vi "RSZVB Start Calibration.vi"(6 "Port 1 (1)":i32=1, 7 "Port 2 (1)":i32=1, 8 "error in (no error)":errorcluster {"code" format="%.0x"}, 9 "Standard (0: Through)":i32(ring) items=["Through"=0, "Open"=1, "Short"=2, "Match"=3, "Symmetric Network"=4, "Attenuation"=5, "Reflect Line"=6, "Line 1"=7, "Line 2"=8, "Offset Short"=9, "Line3"=10, "Sliding Match"=11, "Offset Short 2"=12, "Offset Short 3"=13, "Isolation"=15], 10 "Channel (1)":i32=1, 11 "VISA session":refnum<visa-resource-name>) -> (0 "error out":errorcluster {"code" format="%.0x"}, 3 "dup VISA session":refnum<visa-resource-name>)   [LabVIEW 2011]
doc: "This VI starts a calibration measurement in order to acquire measurement data for the selected standards. The\nstandards are reflection or transmission standards and can be connected to arbitrary analyzer ports.\n\nNote(s):\n\n(1) For some measurements the default set timeout can be insufficient. To set higher timeout use VI RSZVB Set Time Out.vi.\n\n(2) OSHort: Available with firmware version 2.10 and higher.\n\n(3) Line 3 and Sliding Match: Available with firmware version 2.40 and higher.\n\n(4)ISOLation: Available with firmware version 2.78 and higher.\n\nRemote-control command(s):\n[SENSe<Ch>:]CORRection:COLLect[:ACQuire]:SELected THRough | OPEN | SHORt | MATCh | NET | ATT | REFL | LINE | LINE2 | OSHort | LINE3 | SLIDe | OSHORT2 | OSHORT3 | ISOLation,<port_no>[,<port_no>]"
uses:
  _utility/RSZVB Global Data.vi
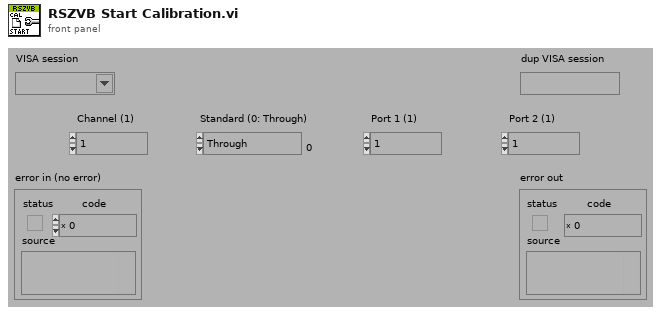
[diagram p1: front panel]
types:
  T1 = cluster{"Error Checking (T: On)":bool, "Installed Options":string[], "Data Valid?":bool, "Ports":i32, "Model":string[], "Option Checking (T: On)":bool}[]
  T2 = cluster{"Error Checking (T: On)":bool, "Installed Options":string[], "Data Valid?":bool, "Ports":i32, "Model":string[], "Option Checking (T: On)":bool}
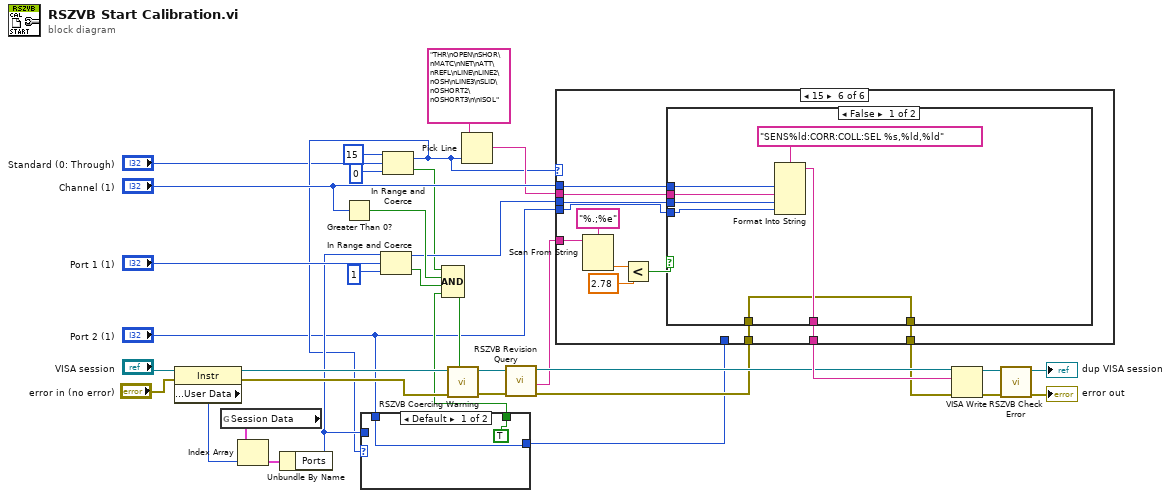
[diagram p0: block diagram]
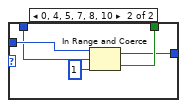
[diagram p2: hidden frame]
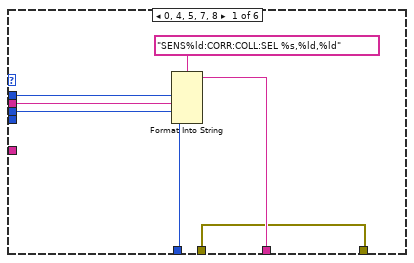
[diagram p3: hidden frame]
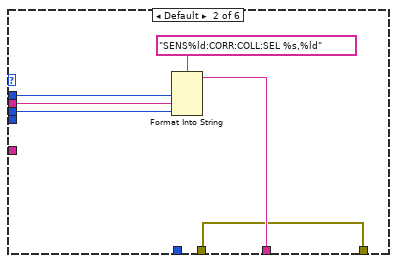
[diagram p4: hidden frame]
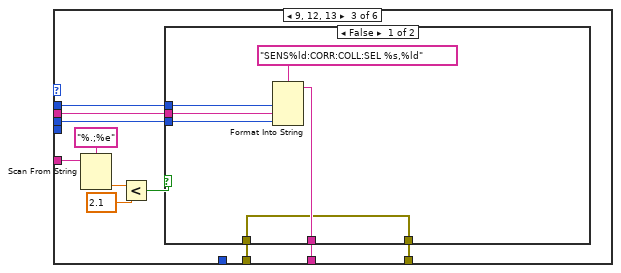
[diagram p5: hidden frame]
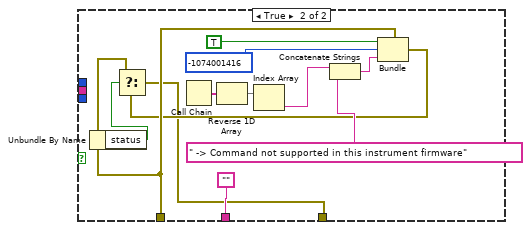
[diagram p6: hidden frame]
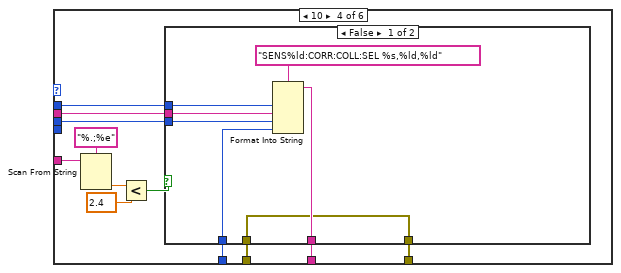
[diagram p7: hidden frame]
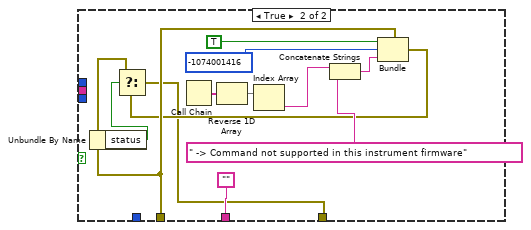
[diagram p8: hidden frame]
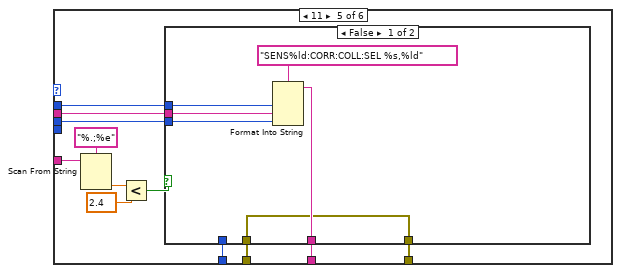
[diagram p9: hidden frame]
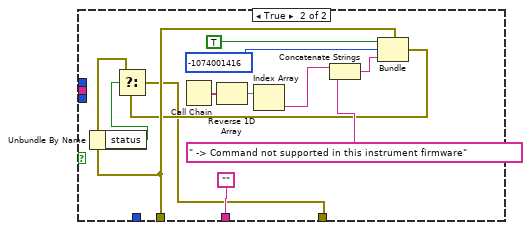
[diagram p10: hidden frame]
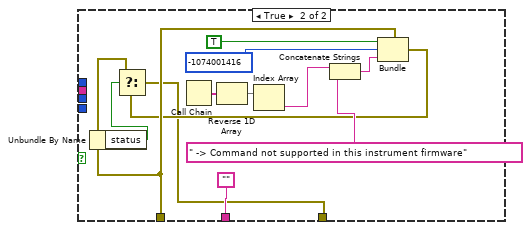
[diagram p11: hidden frame]
diagram:
  n1 = property class="Instr"(reference="VISA session", error in="error in (no error)") -> (reference out=w25:refnum<visa-resource-name>, error out=w26:errorcluster, "General Settings:User Data"=w27:u32)
  n2 = global read "RSZVB Global Data.vi" "Session Data"() -> (w28:T1)
  n3 = Index Array(array=w28, index=w27) -> (element=w29:T2)
  n4 = Unbundle By Name(w29) -> ("Ports"=w8:i32)
  n5 = Greater Than 0?(x="Channel (1)") -> (x > 0?=w30:bool)
  n6 = In Range and Coerce(upper limit=w8, x="Port 1 (1)", lower limit=1) -> (coerced(x)=w14:i32, In Range?=w33:bool)
  n7 = In Range and Coerce(upper limit=15 ("lower limit"), x="Standard (0: Through)", lower limit=0) -> (coerced(x)=w7:i32, In Range?=w13:bool)
  n8 = case shown="Default" w7 {
    tunnel: [TRUE w42] -> w9
    tunnel: w8 -> [_ w41]
    tunnel: [w37 w40] -> w2
    tunnel: "Port 2 (1)" -> [w37 w39]
    frame Default {
    }
    frame 0, 4, 5, 7, 8, 10 {
      n9 = In Range and Coerce(upper limit=w41, x=w39, lower limit=1) -> (coerced(x)=w40:i32, In Range?=w42:bool)
    }
  }
  n10 = Compound Arithmetic op=AND(w13, w30, w33, w9) -> (w32:bool)
  n11 = call "RSZVB Coercing Warning.vi"("In Range?"=w32, "error in (no error)"=w26, "VISA session"=w25) -> ("error out"=w11:errorcluster, "dup VISA session"=w12:refnum<visa-resource-name>)  [unwired: 7 in]
  n12 = Pick Line(multi-line string="THR\nOPEN\nSHOR\nMATC\nNET\nATT\nREFL\nLINE\nLINE2\nOSH\nLINE3\nSLID\nOSHORT2\nOSHORT3\n\nISOL", line index=w7) -> (output string=w15:string)  [unwired: 1 in]
  n13 = call "RSZVB Revision Query.vi"("error in (no error)"=w11, "VISA session"=w12) -> ("error out"=w4:errorcluster, "Instrument Firmware Revision"=w3:string, "dup VISA session"=w10:refnum<visa-resource-name>)  [unwired: 6 in, 1 out]
  n14 = case shown="15" w7 {
    tunnel: [w49 w55 w67 w97 w128 w148] -> w31
    tunnel: "Channel (1)" -> [w48 w54 w66 w96 w127 w154]
    tunnel: w15 -> [w47 w53 w65 w95 w126 w153]
    tunnel: w14 -> [w46 w52 w64 w94 w125 w152]
    tunnel: "Port 2 (1)" -> [_ _ _ _ _ w147]
    tunnel: w3 -> [_ _ w59 w89 w120 w151]
    tunnel: w4 -> [w44 w51 w58 w88 w119 w150]
    tunnel: [w44 w51 w57 w87 w118 w149] -> w5
    tunnel: w2 -> [w45 _ _ w86 w117 _]
    frame 0, 4, 5, 7, 8 {
      n15 = Format Into String(format string="SENS%ld:CORR:COLL:SEL %s,%ld,%ld", w48, w47, w46, w45) -> (resulting string=w49:string)  [unwired: 2 in, 1 out]
    }
    frame Default {
      n16 = Format Into String(format string="SENS%ld:CORR:COLL:SEL %s,%ld", w54, w53, w52) -> (resulting string=w55:string)  [unwired: 2 in, 1 out]
    }
    frame 9, 12, 13 {
      n17 = Scan From String(format string="%.;%e", input string=w59) -> (output 1=w62:dbl)  [unwired: 3 in, 3 out]
      n18 = Less?(x=w62, y=2.1) -> (x < y?=w60:bool)
      n19 = case shown="False" w60 {
        tunnel: [w72 ""] -> w67
        tunnel: w66 -> [w71 _]
        tunnel: w65 -> [w70 _]
        tunnel: w64 -> [w69 _]
        tunnel: w58 -> [w68 w77]
        tunnel: [w68 w74] -> w57
        frame False {
          n20 = Format Into String(format string="SENS%ld:CORR:COLL:SEL %s,%ld", w71, w70, w69) -> (resulting string=w72:string)  [unwired: 2 in, 1 out]
        }
        frame True {
          n21 = Unbundle By Name(w77) -> ("status"=w76:bool)
          n22 = Call Chain() -> (call chain=w81:string[])
          n23 = Reverse 1D Array(array=w81) -> (reversed array=w82:string[])
          n24 = Index Array(array=w82) -> (element=w83:string)  [unwired: 1 in]
          n25 = Concatenate Strings(w83, " -> Command not supported in this instrument firmware" ("string")) -> (w85:string)
          n26 = Bundle(cluster=w77, "status"=TRUE, "code"=-1074001416, "source"=w85) -> (w75:errorcluster)
          n27 = Select(t=w77, s=w76, f=w75) -> (s? t:f=w74:errorcluster)
        }
      }
    }
    frame 10 {
      n28 = Scan From String(format string="%.;%e", input string=w89) -> (output 1=w92:dbl)  [unwired: 3 in, 3 out]
      n29 = Less?(x=w92, y=2.4) -> (x < y?=w90:bool)
      n30 = case shown="False" w90 {
        tunnel: [w103 ""] -> w97
        tunnel: w96 -> [w102 _]
        tunnel: w95 -> [w101 _]
        tunnel: w94 -> [w100 _]
        tunnel: w88 -> [w99 w108]
        tunnel: [w99 w105] -> w87
        tunnel: w86 -> [w98 _]
        frame False {
          n31 = Format Into String(format string="SENS%ld:CORR:COLL:SEL %s,%ld,%ld", w102, w101, w100, w98) -> (resulting string=w103:string)  [unwired: 2 in, 1 out]
        }
        frame True {
          n32 = Unbundle By Name(w108) -> ("status"=w107:bool)
          n33 = Call Chain() -> (call chain=w112:string[])
          n34 = Reverse 1D Array(array=w112) -> (reversed array=w113:string[])
          n35 = Index Array(array=w113) -> (element=w114:string)  [unwired: 1 in]
          n36 = Concatenate Strings(w114, " -> Command not supported in this instrument firmware" ("string")) -> (w116:string)
          n37 = Bundle(cluster=w108, "status"=TRUE, "code"=-1074001416, "source"=w116) -> (w106:errorcluster)
          n38 = Select(t=w108, s=w107, f=w106) -> (s? t:f=w105:errorcluster)
        }
      }
    }
    frame 11 {
      n39 = Scan From String(format string="%.;%e", input string=w120) -> (output 1=w123:dbl)  [unwired: 3 in, 3 out]
      n40 = Less?(x=w123, y=2.4) -> (x < y?=w121:bool)
      n41 = case shown="False" w121 {
        tunnel: [w133 ""] -> w128
        tunnel: w127 -> [w132 _]
        tunnel: w126 -> [w131 _]
        tunnel: w125 -> [w130 _]
        tunnel: w119 -> [w129 w138]
        tunnel: [w129 w135] -> w118
        tunnel: w117 -> [_ _]
        frame False {
          n42 = Format Into String(format string="SENS%ld:CORR:COLL:SEL %s,%ld", w132, w131, w130) -> (resulting string=w133:string)  [unwired: 2 in, 1 out]
        }
        frame True {
          n43 = Unbundle By Name(w138) -> ("status"=w137:bool)
          n44 = Call Chain() -> (call chain=w142:string[])
          n45 = Reverse 1D Array(array=w142) -> (reversed array=w143:string[])
          n46 = Index Array(array=w143) -> (element=w144:string)  [unwired: 1 in]
          n47 = Concatenate Strings(w144, " -> Command not supported in this instrument firmware" ("string")) -> (w146:string)
          n48 = Bundle(cluster=w138, "status"=TRUE, "code"=-1074001416, "source"=w146) -> (w136:errorcluster)
          n49 = Select(t=w138, s=w137, f=w136) -> (s? t:f=w135:errorcluster)
        }
      }
    }
    frame 15 {
      n50 = Scan From String(format string="%.;%e", input string=w151) -> (output 1=w157:dbl)  [unwired: 3 in, 3 out]
      n51 = Less?(x=w157, y=2.78) -> (x < y?=w155:bool)
      n52 = case shown="False" w155 {
        tunnel: [w164 ""] -> w148
        tunnel: w154 -> [w163 _]
        tunnel: w153 -> [w162 _]
        tunnel: w152 -> [w161 _]
        tunnel: w150 -> [w160 w169]
        tunnel: [w160 w166] -> w149
        tunnel: w147 -> [w159 _]
        frame False {
          n53 = Format Into String(format string="SENS%ld:CORR:COLL:SEL %s,%ld,%ld", w163, w162, w161, w159) -> (resulting string=w164:string)  [unwired: 2 in, 1 out]
        }
        frame True {
          n54 = Unbundle By Name(w169) -> ("status"=w168:bool)
          n55 = Call Chain() -> (call chain=w173:string[])
          n56 = Reverse 1D Array(array=w173) -> (reversed array=w174:string[])
          n57 = Index Array(array=w174) -> (element=w175:string)  [unwired: 1 in]
          n58 = Concatenate Strings(w175, " -> Command not supported in this instrument firmware" ("string")) -> (w177:string)
          n59 = Bundle(cluster=w169, "status"=TRUE, "code"=-1074001416, "source"=w177) -> (w167:errorcluster)
          n60 = Select(t=w169, s=w168, f=w167) -> (s? t:f=w166:errorcluster)
        }
      }
    }
  }
  n61 = VISA Write(VISA resource name=w10, write buffer=w31, error in (no error)=w5) -> (VISA resource name out=w34:refnum<visa-resource-name>, error out=w35:errorcluster)  [unwired: 1 out]
  n62 = call "RSZVB Check Error.vi"("error in (no error)"=w35, "VISA session"=w34) -> ("error out"=→"error out":errorcluster, "dup VISA session"=→"dup VISA session":refnum<visa-resource-name>)  [unwired: 8 in]
